vi "subReduceBuildOrder.vi"(11 "Ordering map":T1) -> (0 "error out":errorcluster, 3 "Raw build order":refnum<class "ProjectItem.lvclass">[](array[class]))   [LabVIEW 2019, in "SolutionBuilder.lvlib" / "SolutionBuilder.lvclass"]
uses:
  SolutionBuilder.lvclass
  ProjectItem/ProjectItem.lvclass
  OrderingMap.ctl
  ProjectItem/ProjectItem.lvclass/ProjectItem.ctl
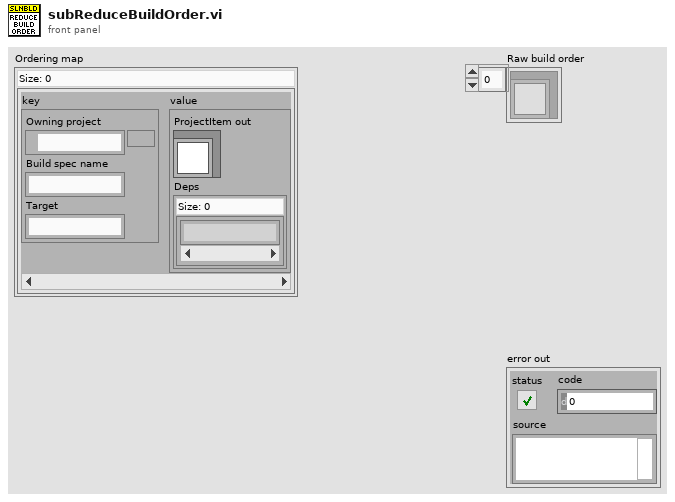
[diagram p1: front panel]
types:
  T1 = typedef "SolutionBuilder.lvlib/SolutionBuilder.lvclass/OrderingMap.ctl" = map{cluster{"Owning project":path, "Build spec name":string, "Target":string}, cluster{"ProjectItem out":refnum<class "ProjectItem.lvclass">, "Deps":set{string}}}
  T2 = cluster{"Owning project":path, "Build spec name":string, "Target":string}
  T3 = cluster{"ProjectItem out":refnum<class "ProjectItem.lvclass">, "Deps":set{string}}
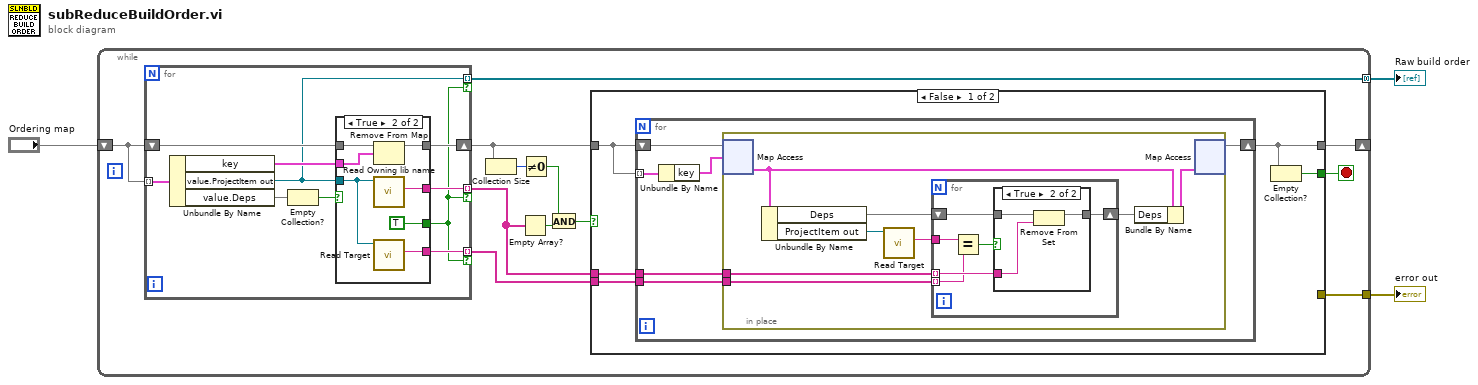
[diagram p0: block diagram]
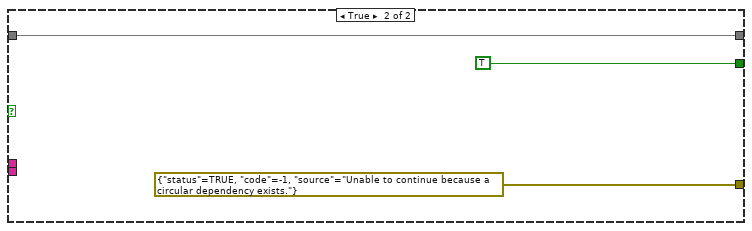
[diagram p4: hidden frame]
diagram:
  n1 = while {
    shift-right: [w13] -> _
    shift-left: "Ordering map" -> [w15]
    tunnel: [w5] -> w3 mode=concatenating
    tunnel: [w6] -> w1
    stop <- w14 stop-if-true
    n2 = for {
      tunnel: w15 -> [w21] mode=indexing
      shift-right: [w24] -> w12
      shift-left: w15 -> [w25]
      tunnel: [w23] -> w11 mode=indexing if=w16
      tunnel: [w19] -> w5 mode=indexing if=w16
      tunnel: [w17] -> w4 mode=indexing if=w16
      n3 = Unbundle By Name(w21) -> ("key"=w20:T2, "value.ProjectItem out"=w19:refnum<class "ProjectItem.lvclass">, "value.Deps"=w18:set{string})
      n4 = Empty Collection?(1:w18) -> (0:w22:bool)
      n5 = case shown="True" w22 {
        tunnel: w25 -> [w26 w33]
        tunnel: [w26 w32] -> w24
        tunnel: w20 -> [_ w31]
        tunnel: [_ w27] -> w23
        tunnel: [_ TRUE] -> w16
        tunnel: w19 -> [_ w28]
        tunnel: [_ w29] -> w17
        frame False {
        }
        frame True {
          n6 = Remove From Map(10:w31, 11:w33) -> (3:w32:T1)  [unwired: 2 out]
          n7 = call "Read Owning lib name.vi"("ProjectItem in"=w28) -> ("Owning lib name"=w27:string)  [unwired: 9 in, 1 out]
          n8 = call "Read Target.vi"("ProjectItem in"=w28) -> ("Target"=w29:string)  [unwired: 9 in, 1 out]
        }
      }
    }
    n9 = Collection Size(1:w12) -> (0:w10:i32)
    n10 = Empty Array?(array=w11) -> (empty?=w9:bool)
    n11 = Not Equal To 0?(x=w10) -> (x != 0?=w8:bool)
    n12 = And(x=w8, y=w9) -> (x .and. y?=w7:bool)
    n13 = case shown="False" w7 {
      tunnel: [w38 TRUE ("empty?")] -> w14
      tunnel: w12 -> [w37 w65]
      tunnel: w11 -> [w36 _]
      tunnel: [w35 w65] -> w13
      tunnel: [_ errorcluster {"status"=TRUE, "code"=-1, "source"="Unable to continue because a circular dependency exists."} ("error IO")] -> w6
      tunnel: w4 -> [w34 _]
      frame False {
        n14 = for {
          shift-right: [w42] -> w35
          shift-left: w37 -> [w44]
          tunnel: w37 -> [w41] mode=indexing
          tunnel: w36 -> [w43]
          tunnel: w34 -> [w39]
          n15 = Unbundle By Name(w41) -> ("key"=w40:T2)
          n16 = in-place {
            in-place-border: w43 -> [w52]
            in-place-border: w39 -> [w48]
            n17 = in-place-map #1(w44, w40) -> (w47:T3)  [unwired: 1 in, 1 out]
            n18 = Unbundle By Name(w47) -> ("Deps"=w51:set{string}, "ProjectItem out"=w46:refnum<class "ProjectItem.lvclass">)
            n19 = call "Read Target.vi"("ProjectItem in"=w46) -> ("Target"=w45:string)  [unwired: 9 in, 1 out]
            n20 = for {
              tunnel: w52 -> [w57] mode=indexing
              shift-right: [w56] -> w50
              shift-left: w51 -> [w58]
              tunnel: w48 -> [w54] mode=indexing
              tunnel: w45 -> [w55]
              n21 = Equal?(x=w55, y=w54) -> (x = y?=w53:bool)
              n22 = case shown="True" w53 {
                tunnel: w58 -> [w59 w62]
                tunnel: w57 -> [_ w61]
                tunnel: [w59 w60] -> w56
                frame False {
                }
                frame True {
                  n23 = Remove From Set(10:w61, 11:w62) -> (3:w60:set{string})  [unwired: 1 out]
                }
              }
            }
            n24 = Bundle By Name(cluster=w47, "Deps"=w50) -> (w49:T3)
            n25 = in-place-map #1(w49) -> (w42:T1)  [unwired: 1 in, 2 out]
          }
        }
        n26 = Empty Collection?(1:w35) -> (0:w38:bool)
      }
      frame True {
      }
    }
  }
  "Raw build order" <- w3
  "error out" <- w1
